vi "VCS Open Device Dlg.vi"(8 "error in (no error)":errorcluster) -> (0 "error out":errorcluster, 3 "keyHandle out":u32)   [LabVIEW 2017, in "maxonEPOS.lvlib"]
doc: "<B>VCS Open Device Dlg</B> registers available interfaces (CAN, USB and RS232) with which the EPOS family can be operated and opened the selected interface for communication."
uses:
  Examples/maxonEPOS.lvlib
  Resources/EposCmd.dll
  SSI_Tool/InstrumentsInterfaces/Motordriver/maxon EPOS/Resources/EposCmd64.dll
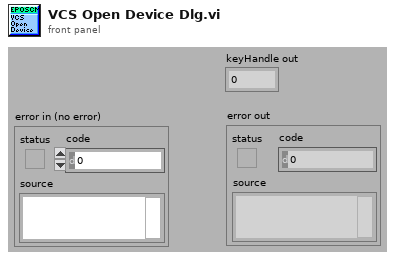
[diagram p1: front panel]
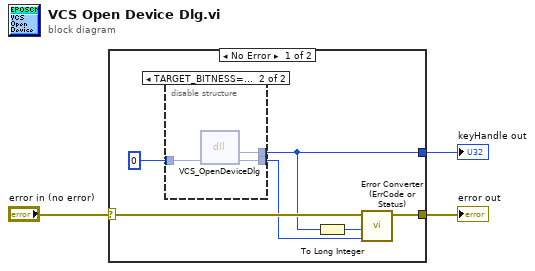
[diagram p0: block diagram]
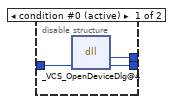
[diagram p2: hidden frame]
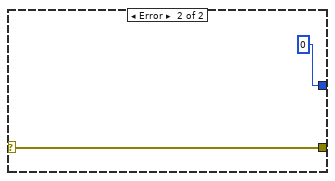
[diagram p3: hidden frame]
diagram:
  n1 = case shown="No Error" "error in (no error)" {
    selector: "error in (no error)" -> [w9 w17]
    tunnel: [w8 w17] -> w2
    tunnel: [w4 u32 0] -> w1
    frame No Error {
      n2 = disable-structure shown="TARGET_BITNESS==64" {
        disable-tunnel: [w12 w15] -> w7
        disable-tunnel: u32 0 ("pErrorCode") -> [w11 w14]
        disable-tunnel: [w10 w13] -> w4
        frame condition #0 (active) {
          n3 = dll-call lib="C:/workspace/project/scancon/sw/SSI_Tool/InstrumentsInterfaces/Motordriver/maxon EPOS/Resources/EposCmd.dll" fn="_VCS_OpenDeviceDlg@4"("pErrorCode"=w11) -> ("return type"=w10:u32, "pErrorCode"=w12:u32)  [unwired: 3 in, 2 out]
        }
        frame condition #1 {
          n4 = dll-call lib="C:/Sources/LabView/maxon EPOS/Resources/EposCmd64.dll" fn="VCS_OpenDeviceDlg"("pErrorCode"=w14) -> ("return type"=w13:u32, "pErrorCode"=w15:u32)  [unwired: 3 in, 2 out]
        }
      }
      n5 = To Long Integer(number=w4) -> (32bit integer=w5:i32)
      n6 = call "Error Converter (ErrCode or Status).vi"("error code"=w7, "return type"=w5, "error in (no error)"=w9) -> ("error out"=w8:errorcluster)  [unwired: 7 in]
    }
    frame Error {
    }
  }
  "error out" <- w2
  "keyHandle out" <- w1
